vi "Get Scheme.vi"(8 "error in (no error)":errorcluster, 10 "Theme":u16(ring) items=["Light Theme", "Light Medium Contrast", "Light High Contrast", "Dark Theme", "Dark Medium Contrast", "Dark High Constrast"], 11 "Material Theme in":refnum<class "Material Theme.lvclass">) -> (0 "error out":errorcluster, 2 "Material-Scheme":refnum<class "Material-Scheme.lvclass">, 3 "Material Theme out":refnum<class "Material Theme.lvclass">)   [LabVIEW 2021, in "TSC Material Theme.lvlib" / "Material Theme.lvclass"]
doc: "Get the defined scheme from the loaded theme\n\n<b>Code Developed By:</b> +\nDaniel Coons +\nTechnology Service Corporation +\nwww.tsc.com/atcs"
uses:
  Material Theme.lvclass
  Material-Scheme/Material-Scheme.lvclass
  Material Theme.lvclass/Material Theme.ctl
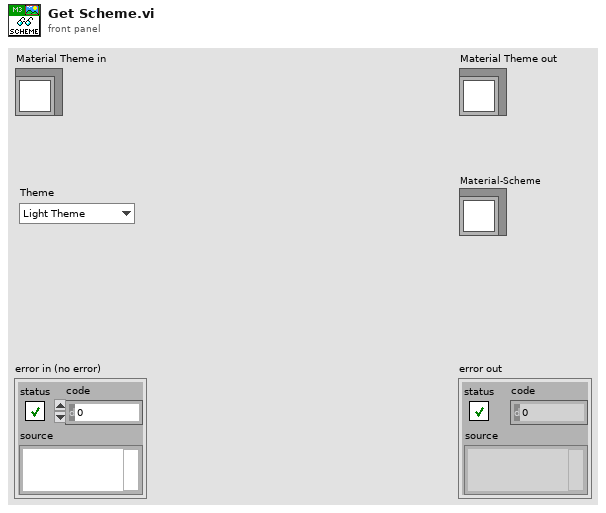
[diagram p1: front panel]
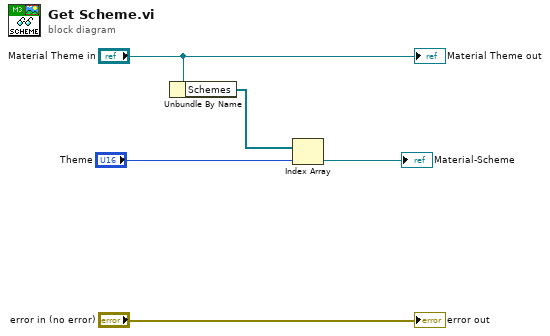
[diagram p0: block diagram]
diagram:
  n1 = Unbundle By Name("Material Theme in") -> ("Schemes"=w3:refnum<class "Material-Scheme.lvclass">[])
  n2 = Index Array(array=w3, index="Theme") -> (element=→"Material-Scheme":refnum<class "Material-Scheme.lvclass">)
  "error out" <- "error in (no error)"
  "Material Theme out" <- "Material Theme in"
